vi "getHardwareRevision.vi"(8 "error in (no error)":errorcluster, 11 "IDeviceInfo in":refnum<class "IDeviceInfo.lvclass">) -> (0 "error out":errorcluster, 2 "HardwareRevision out":string, 3 "IDeviceInfo out":refnum<class "IDeviceInfo.lvclass">)   [LabVIEW 2022 SP3, in "openDAQ.lvlib" / "IBaseObject.lvlib" / "IPropertyObject.lvlib" / "IDeviceInfo.lvlib" / "IDeviceInfo.lvclass"]
uses:
  <instrlib>/openDAQ/Public/Classes/IDeviceInfo/IDeviceInfo.lvclass
  <instrlib>/openDAQ/Public/Classes/IDeviceInfo/IDeviceInfo.lvclass/IDeviceInfo.ctl
  <instrlib>/openDAQ/Public/Classes/daqCoreTypes/IString/IString.lvclass
  <instrlib>/openDAQ/Binaries/Windows/x86/copendaq32.dll
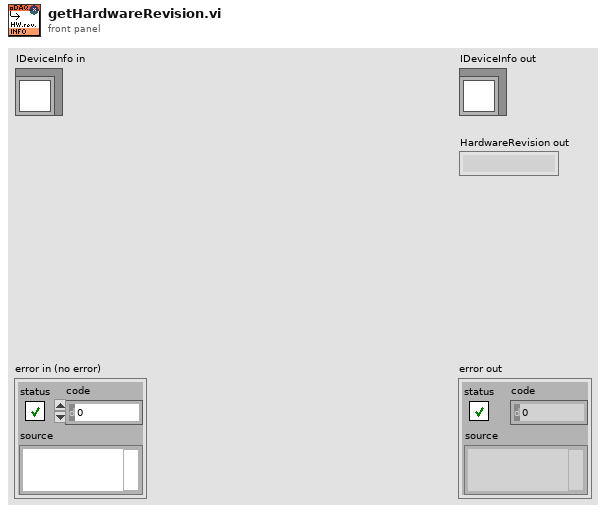
[diagram p1: front panel]
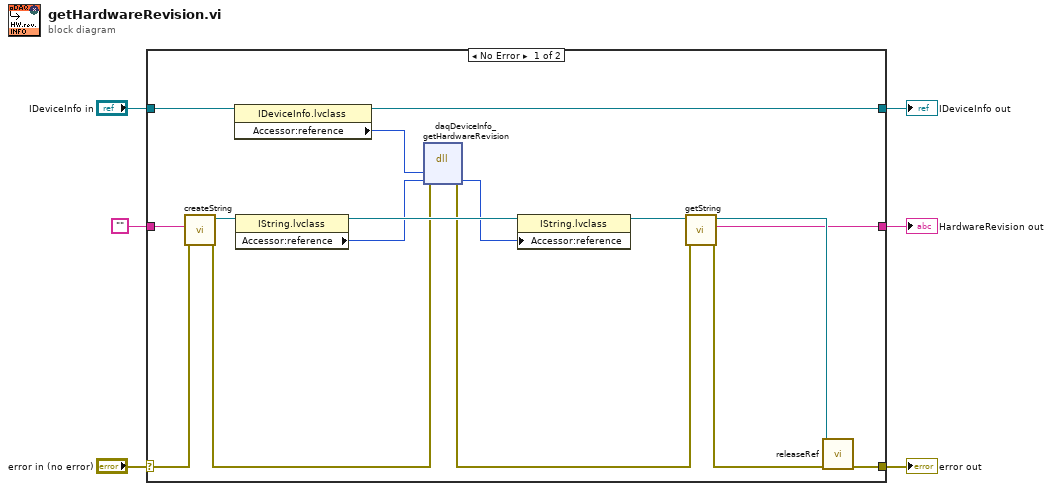
[diagram p0: block diagram]
diagram:
  n1 = case shown="No Error" "error in (no error)" {
    selector: "error in (no error)" -> [w8 w25]
    tunnel: [w14 w25] -> w5
    tunnel: [w18 w24] -> w3
    tunnel: "IDeviceInfo in" -> [w20 w24]
    tunnel: "" -> [w17 w23]
    tunnel: [w9 w23] -> w1
    frame No Error {
      n2 = call <instrlib>:"createString.vi"("error in (no error)"=w8, "String"=w17) -> ("error out"=w7:errorcluster, "IString out"=w21:refnum<class "IString.lvclass">)  [unwired: 8 in]
      n3 = property class="IDeviceInfo.lvclass"(reference=w20) -> (reference out=w18:refnum<class "IDeviceInfo.lvclass">, "Accessor:reference"=w19:i64)  [unwired: 1 in, 1 out]
      n4 = property class="IString.lvclass"(reference=w21) -> (reference out=w22:refnum<class "IString.lvclass">, "Accessor:reference"=w16:i64)  [unwired: 1 in, 1 out]
      n5 = dll-call lib="C:/Program Files (x86)/National Instruments/LabVIEW 2022/instr.lib/openDAQ/Binaries/Windows/x86/copendaq*.*" fn="daqDeviceInfo_getHardwareRevision"(error in=w7, "deviceInfo"=w19, "hardwareRevision"=w16) -> (error out=w11:errorcluster, "hardwareRevision"=w15:i64)  [unwired: 4 in, 1 out]
      n6 = property class="IString.lvclass"(reference=w22, "Accessor:reference"=w15) -> (reference out=w13:refnum<class "IString.lvclass">)  [unwired: 1 in, 1 out]
      n7 = call <instrlib>:"getString.vi"("error in (no error)"=w11, "IString in"=w13) -> ("error out"=w10:errorcluster, "String out"=w9:string, "IString out"=w12:refnum<class "IString.lvclass">)  [unwired: 7 in]
      n8 = call-dynamic "releaseRef.vi"("error in (no error)"=w10, "IBaseObject in"=w12) -> ("error out"=w14:errorcluster)  [unwired: 9 in]
    }
    frame Error {
    }
  }
  "error out" <- w5
  "IDeviceInfo out" <- w3
  "HardwareRevision out" <- w1
